vi "Framework Listener Sobot.vi"() -> ()   [LabVIEW 2017]
uses:
  TypeDefinitions/TCP Commands.ctl
  TypeDefinitions/TCP Cluster.ctl
panel:
  out "Send":T1={"Datatype"=enum."Message", "String"="Send to sobot"}
  out "Receive":T1={"Datatype"=enum."Message", "String"="Send to sobot"}
  in  "Button 2":bool
  in  "stop":bool
  in  "Button 1":bool
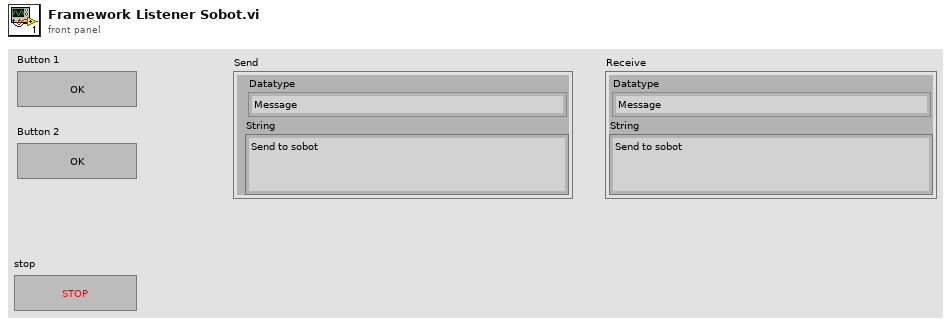
[diagram p1: front panel]
types:
  T1 = typedef "TCP Cluster.ctl" = cluster{"Datatype":T2, "String":string}
  T2 = typedef "TCP Commands.ctl" = enum16{"Message", "Stop", "Command"}
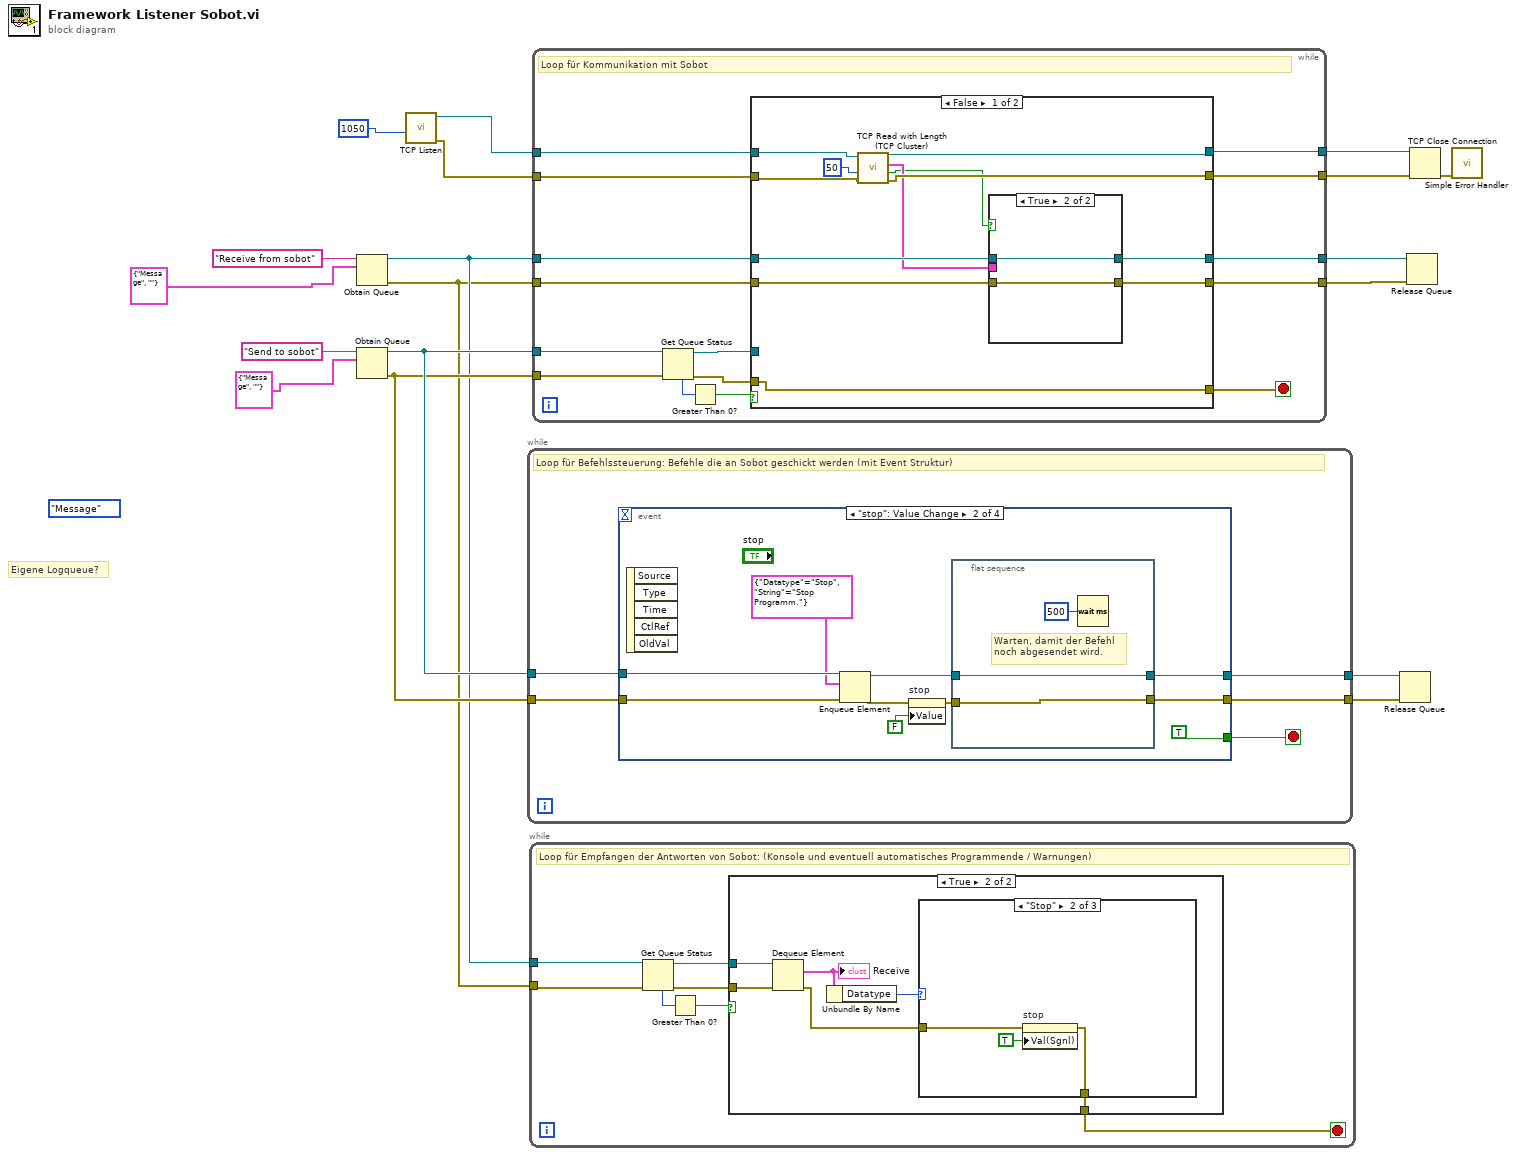
[diagram p0: block diagram]
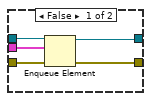
[diagram p5: hidden frame]
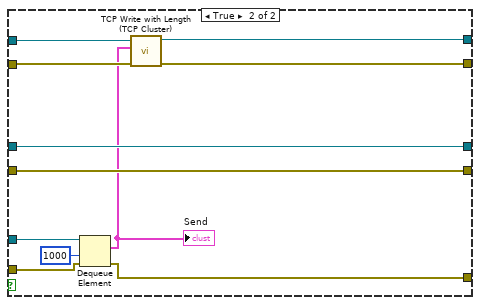
[diagram p6: hidden frame]
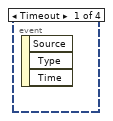
[diagram p7: hidden frame]
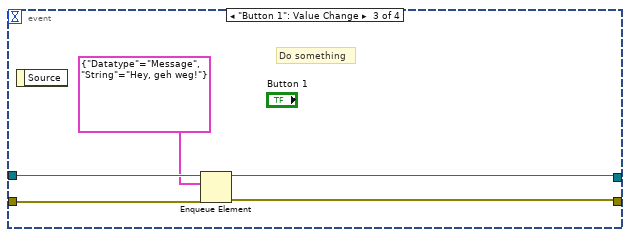
[diagram p8: hidden frame]
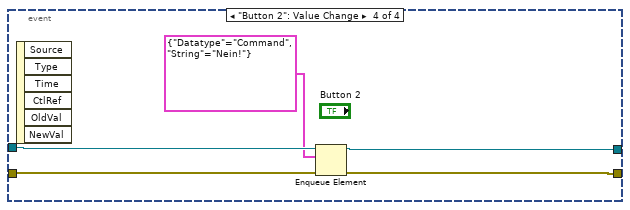
[diagram p9: hidden frame]
diagram:
  (unwired) TCP_Commands."Message"
  # "Eigene Logqueue?"
  n1 = Obtain Queue(name (unnamed)="Receive from sobot", element data type=T1 {"Datatype"=enum."Message", "String"=""}) -> (queue out=w9:refnum<queue>, error out=w8:errorcluster)  [unwired: 3 in, 1 out]
  n2 = Obtain Queue(name (unnamed)="Send to sobot", element data type=T1 {"Datatype"=enum."Message", "String"=""}) -> (queue out=w17:refnum<queue>, error out=w14:errorcluster)  [unwired: 3 in, 1 out]
  n3 = call <vilib>:"TCP Listen.vi"("timeout ms (wait forever: -1)"=u16 1050 ("remote port or service name")) -> ("error out"=w2:errorcluster, "connection ID"=w1:refnum<k5>)  [unwired: 6 in, 3 out]
  n4 = while {
    tunnel: w17 -> [w22]
    tunnel: [w21] -> w16
    tunnel: [w20] -> w15
    tunnel: w14 -> [w19]
    stop <- w23 stop-if-true
    # "Loop für Befehlssteuerung: Befehle die an Sobot geschickt werden (mit Event Struktur)"
    n5 = event shown="[1] \"stop\": Value Change" {
      selector: _ -> [_ _ _ _]
      dyn-events: _ -> [_ _ _ _]
      timeout: _ -> [_ _ _ _]
      tunnel: [_ TRUE _ _] -> w23
      tunnel: w22 -> [_ w32 w41 w46]
      tunnel: [_ w28 w38 w45] -> w21
      tunnel: [_ w25 w39 w44] -> w20
      tunnel: w19 -> [_ w31 w40 w43]
      event Timeout {
        n6 = event-data() -> ()  [unwired: 1 in, 3 out]
      }
      event "stop": Value Change {
        n7 = event-data() -> ()  [unwired: 1 in, 5 out]
        n8 = Enqueue Element(queue=w32, element=T1 {"Datatype"=enum."Stop", "String"="Stop Programm."}, error in (no error)=w31) -> (queue out=w29:refnum<queue>, error out=w27:errorcluster)  [unwired: 1 in, 1 out]
        n9 = property on="stop" class="Bool (strict)"(error in=w27, "Value"=FALSE ("stop")) -> (error out=w24:errorcluster)  [unwired: 1 in, 1 out]
        n10 = flat-sequence {
          tunnel: w29 -> [w36]
          tunnel: [w36] -> w28
          tunnel: [w34] -> w25
          tunnel: w24 -> [w34]
          frame #0 {
            # "Warten, damit der Befehl\nnoch abgesendet wird."
            n11 = Wait (ms)(milliseconds to wait=u32 500) -> ()  [unwired: 1 out]
          }
        }
      }
      event "Button 1": Value Change {
        # "Do something"
        n12 = event-data() -> ()  [unwired: 1 in, 1 out]
        n13 = Enqueue Element(queue=w41, element=T1 {"Datatype"=enum."Message", "String"="Hey, geh weg!"}, error in (no error)=w40) -> (queue out=w38:refnum<queue>, error out=w39:errorcluster)  [unwired: 1 in, 1 out]
      }
      event "Button 2": Value Change {
        n14 = event-data() -> ()  [unwired: 1 in, 6 out]
        n15 = Enqueue Element(queue=w46, element=T1 {"Datatype"=enum."Command", "String"="Nein!"}, error in (no error)=w43) -> (queue out=w45:refnum<queue>, error out=w44:errorcluster)  [unwired: 1 in, 1 out]
      }
    }
  }
  n16 = while {
    tunnel: w9 -> [w52]
    tunnel: w8 -> [w51]
    stop <- w47 stop-if-true
    # "Loop für Empfangen der Antworten von Sobot: (Konsole und eventuell automatisches Programmende / Warnungen)"
    n17 = Get Queue Status(queue=w52, error in (no error)=w51) -> (queue out=w49:refnum<queue>, error out=w48:errorcluster, # elements in queue=w53:i32)  [unwired: 1 in, 5 out]
    n18 = Greater Than 0?(x=w53) -> (x > 0?=w50:bool)
    n19 = case shown="True" w50 {
      tunnel: w49 -> [_ w60]
      tunnel: w48 -> [w54 w59]
      tunnel: [w54 w55] -> w47
      frame False {
      }
      frame True {
        n20 = Dequeue Element(queue=w60, error in (no error)=w59) -> (element=w58:T1, error out=w56:errorcluster)  [unwired: 1 in, 2 out]
        "Receive" <- w58
        n21 = Unbundle By Name(w58) -> ("Datatype"=w57:T2)
        n22 = case shown="\"Stop\"" w57 {
          tunnel: w56 -> [w61 w63 w65]
          tunnel: [w61 w62 w65] -> w55
          frame "Message", Default {
          }
          frame "Stop" {
            n23 = property on="stop" class="Bool (strict)"(error in=w63, "Val(Sgnl)"=TRUE ("Value (Signaling)")) -> (error out=w62:errorcluster)  [unwired: 1 in, 1 out]
          }
          frame "Command" {
          }
        }
      }
    }
  }
  n24 = while {
    tunnel: w17 -> [w79]
    tunnel: w14 -> [w77]
    tunnel: w1 -> [w73]
    tunnel: w2 -> [w72]
    tunnel: [w71] -> w12
    tunnel: [w70] -> w11
    tunnel: w9 -> [w69]
    tunnel: w8 -> [w68]
    tunnel: [w67] -> w6
    tunnel: [w66] -> w7
    stop <- w80 stop-if-true
    # "Loop für Kommunikation mit Sobot"
    n25 = Get Queue Status(queue=w79, error in (no error)=w77) -> (queue out=w78:refnum<queue>, error out=w76:errorcluster, # elements in queue=w75:i32)  [unwired: 1 in, 5 out]
    n26 = Greater Than 0?(x=w75) -> (x > 0?=w74:bool)
    n27 = case shown="False" w74 {
      tunnel: [w92 w110] -> w80
      tunnel: w78 -> [_ w108]
      tunnel: w76 -> [w92 w107]
      tunnel: w73 -> [w87 w104]
      tunnel: w72 -> [w86 w103]
      tunnel: [w84 w102] -> w70
      tunnel: [w83 w101] -> w71
      tunnel: w69 -> [w91 w106]
      tunnel: w68 -> [w90 w105]
      tunnel: [w89 w106] -> w66
      tunnel: [w88 w105] -> w67
      frame False {
        n28 = call "TCP Read with Length (TCP Cluster).vi"("error in (no error)"=w86, "Timeout"=50, "connection ID"=w87) -> ("error out"=w84:errorcluster, "Timeout?"=w81:bool, "TCP Cluster"=w82:T1, "connection ID out"=w83:refnum<k5>)  [unwired: 5 in]
        n29 = case shown="True" w81 {
          tunnel: w91 -> [w97 w99]
          tunnel: w90 -> [w96 w98]
          tunnel: w82 -> [w95 _]
          tunnel: [w94 w99] -> w89
          tunnel: [w93 w98] -> w88
          frame False {
            n30 = Enqueue Element(queue=w97, element=w95, error in (no error)=w96) -> (queue out=w94:refnum<queue>, error out=w93:errorcluster)  [unwired: 1 in, 1 out]
          }
          frame True {
          }
        }
      }
      frame True {
        n31 = Dequeue Element(queue=w108, timeout in ms (-1)=1000, error in (no error)=w107) -> (element=w100:T1, error out=w110:errorcluster)  [unwired: 2 out]
        "Send" <- w100
        n32 = call "TCP Write with Length (TCP Cluster).vi"("error in (no error)"=w103, 10:w100, "connection ID"=w104) -> ("error out"=w102:errorcluster, "connection ID out"=w101:refnum<k5>)  [unwired: 7 in]
      }
    }
  }
  n33 = Release Queue(queue=w16, error in (no error)=w15) -> ()  [unwired: 1 in, 3 out]
  n34 = Release Queue(queue=w7, error in (no error)=w6) -> ()  [unwired: 1 in, 3 out]
  n35 = TCP Close Connection(connection ID=w12, error in (no error)=w11) -> (error out=w13:errorcluster)  [unwired: 1 in, 1 out]
  n36 = call <vilib>:"Simple Error Handler.vi"("error in (no error)"=w13) -> ()  [unwired: 4 in, 5 out]
